vi "Draw Shapes.vi"(0 "Picture in":refnum<vi>, 1 "Commands":cluster{"Time (s)":dbl, T2, "Enabled":bool}[](array[cluster]), 2 "dt array":dbl[](array[numeric]), 3 "Sample Period (s)":dbl=0.02, 5 "Points":cluster{"x":dbl, "y":dbl, "th":dbl}[](array[cluster]), 7 "new picture in":picture, 9 "Path Type":T1, 11 "Results":T5, 12 "Output Point":T4, 14 "Path Points":cluster{"x":dbl, "y":dbl}[](array[cluster])) -> (4 "new picture out":picture)   [LabVIEW 2025]
uses:
  Types/Single Cmd Info.ctl
  <vilib>/picture/picture.llb/imagedata.ctl
  Types/Path Type.ctl
  Global Settings.vi
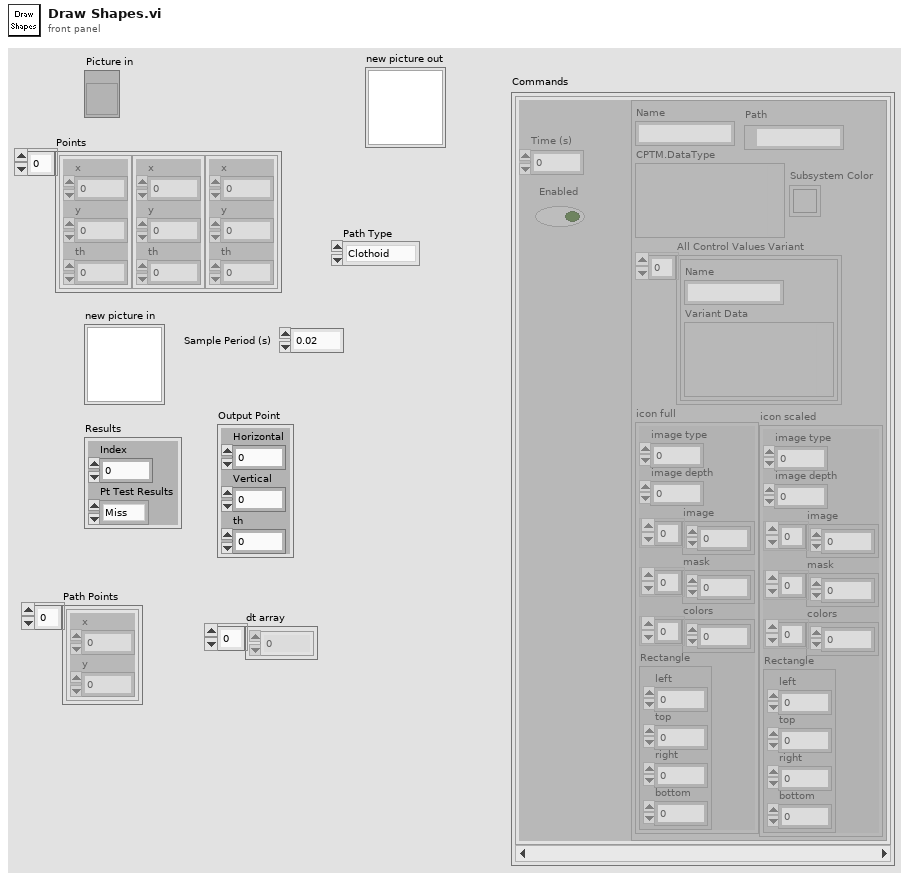
[diagram p1: front panel]
types:
  T1 = typedef "Path Type.ctl" = enum16{"Clothoid", "Bezier", "Choreo"}
  T2 = typedef "Single Cmd Info.ctl" = cluster{"Name":string, "CPTM.DataType":variant, "All Control Values Variant":cluster{"Name":string, "Variant Data":variant}[], "icon full":T3, "icon scaled":T3, "Path":path, "Subsystem Color":u32}
  T3 = typedef "imagedata.ctl" = cluster{"image type":i32, "image depth":i32, "image":u8[], "mask":u8[], "colors":u32[], "Rectangle":cluster{"left":i16, "top":i16, "right":i16, "bottom":i16}}
  T4 = cluster{"Horizontal":dbl, "Vertical":dbl, "th":dbl}
  T5 = cluster{"Index":i32, "Pt Test Results":enum16{"Miss", "Rect Hit", "Arrow Hit"}}
  T6 = typedef "LVPositionTypeDef.ctl" = cluster{"Left":i32, "Top":i32}
  T7 = typedef "LVBoundsTypeDef.ctl" = cluster{"Width":u32, "Height":u32}
  T8 = cluster{"left":i16, "top":i16, "right":i16, "bottom":i16}
  T9 = cluster{"Horizontal":dbl, "Vertical":dbl, "Horizontal":dbl, "Vertical":dbl}
  T10 = cluster{i32, "Pt Test Results":enum16{"Miss", "Rect Hit", "Arrow Hit"}}
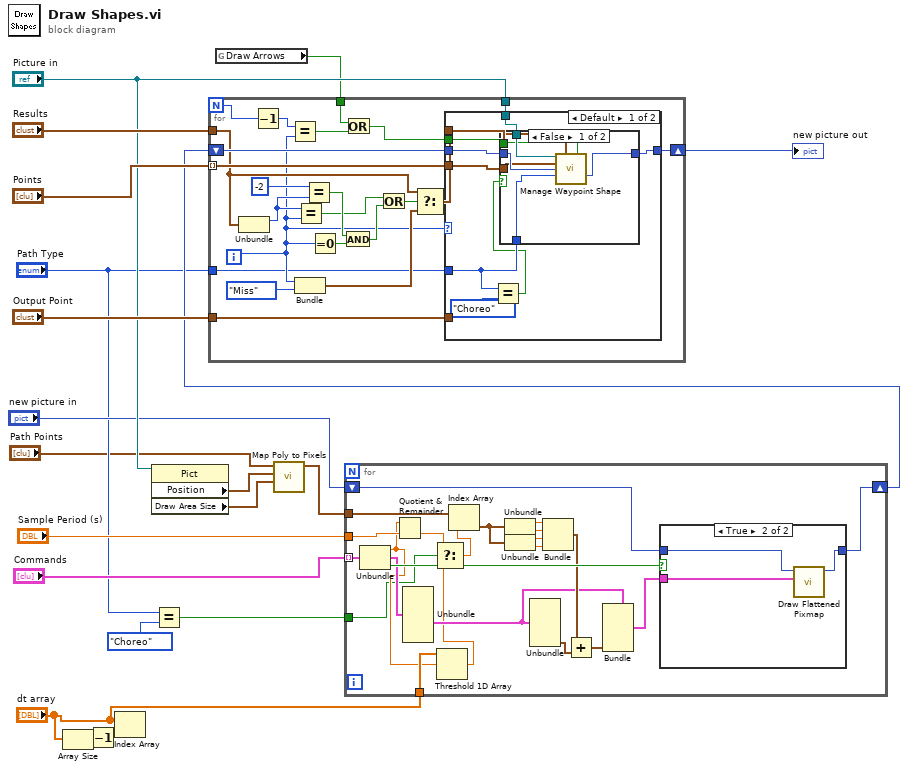
[diagram p0: block diagram]
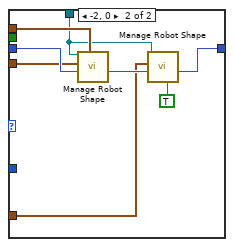
[diagram p4: hidden frame]
diagram:
  n1 = Array Size(array="dt array") -> (size(s)=w4:i32)
  n2 = Decrement(x=w4) -> (x-1=w3:i32)
  n3 = Index Array(array="dt array", index=w3) -> ()  [unwired: 1 out]
  n4 = property on="Property Node" class="Pict"(reference="Picture in") -> ("Position"=w14:T6, "Draw Area Size"=w15:T7)  [unwired: 1 in, 2 out]
  n5 = Equal?(x="Path Type", y=Path_Type."Choreo") -> (x = y?=w1:bool)
  n6 = global read "Global Settings.vi" "Draw Arrows"() -> (w8:bool)
  n7 = call "Map Poly to Pixels.vi"("Draw Area Size"=w15, "Position"=w14, "Coords"="Path Points") -> ("Coords"=w13:cluster{"Horizontal":dbl, "Vertical":dbl}[])  [unwired: 8 in]
  n8 = for {
    shift-right: [w38] -> w10
    shift-left: "new picture in" -> [w40]
    tunnel: "Commands" -> [w43] mode=indexing
    tunnel: w13 -> [w42]
    tunnel: "Sample Period (s)" -> [w41]
    tunnel: "dt array" -> [w26]
    tunnel: w1 -> [w24]
    n9 = Unbundle(w43) -> ("Time (s)"=w25:dbl, w36:T2, "Enabled"=w39:bool)
    n10 = Quotient & Remainder(x=w25, y=w41) -> (floor(x/y)=w23:dbl)  [unwired: 1 out]
    n11 = Unbundle(w36) -> ("icon scaled"=w28:T3)  [unwired: 6 out]
    n12 = Threshold 1D Array(2:w25, 3:w26) -> (0:w22:dbl)  [unwired: 1 in]
    n13 = Select(t=w22, s=w24, f=w23) -> (s? t:f=w21:dbl)
    n14 = Index Array(array=w42, index=w21) -> (element=w27:cluster{"Horizontal":dbl, "Vertical":dbl})
    n15 = Unbundle(w27) -> ("Horizontal"=w35:dbl, "Vertical"=w34:dbl)
    n16 = Unbundle(w27) -> ("Horizontal"=w33:dbl, "Vertical"=w32:dbl)
    n17 = Unbundle(w28) -> ("Rectangle"=w30:T8)  [unwired: 5 out]
    n18 = Bundle("Horizontal"=w35, "Vertical"=w34, "Horizontal"=w33, "Vertical"=w32) -> (w29:T9)  [unwired: 1 in]
    n19 = Add(x=w29, y=w30) -> (x+y=w37:cluster{dbl, dbl, dbl, dbl})
    n20 = Bundle(cluster=w28, "Rectangle"=w37) -> (w31:T3)  [unwired: 5 in]
    n21 = case shown="True" w39 {
      tunnel: [w44 w45] -> w38
      tunnel: w40 -> [w44 w46]
      tunnel: w31 -> [_ w47]
      frame False {
      }
      frame True {
        n22 = call <vilib>:"Draw Flattened Pixmap.vi"("image data"=w47, "picture"=w46) -> ("new picture"=w45:picture)  [unwired: 7 in]
      }
    }
  }
  n23 = for {
    N -> [w55]
    tunnel: "Points" -> [w70] mode=indexing
    shift-right: [w69] -> w9
    shift-left: w10 -> [w68]
    tunnel: "Picture in" -> [w67]
    tunnel: "Results" -> [w64]
    tunnel: "Output Point" -> [w52]
    tunnel: w8 -> [w49]
    tunnel: "Path Type" -> [w48]
    i -> [w53]
    n24 = Unbundle(w64) -> ("Index"=w60:i32)  [unwired: 1 out]
    n25 = Decrement(x=w55) -> (x-1=w54:i32)
    n26 = Equal?(x=w54, y=w53) -> (x = y?=w51:bool)
    n27 = Bundle(w53, "Pt Test Results"=enum16{"Miss", "Rect Hit", "Arrow Hit"}."Miss") -> (w65:T10)  [unwired: 1 in]
    n28 = Equal?(x=w60, y=w53) -> (x = y?=w57:bool)
    n29 = Equal?(x=-2, y=w60) -> (x = y?=w59:bool)
    n30 = Equal To 0?(x=w53) -> (x = 0?=w62:bool)
    n31 = And(x=w59, y=w62) -> (x .and. y?=w58:bool)
    n32 = Or(x=w49, y=w51) -> (x .or. y?=w50:bool)
    n33 = Or(x=w57, y=w58) -> (x .or. y?=w56:bool)
    n34 = Select(t=w64, s=w56, f=w65) -> (s? t:f=w66:T5)
    n35 = case shown="Default" w53 {
      tunnel: w70 -> [w75 w88]
      tunnel: [w78 w92] -> w69
      tunnel: w68 -> [w79 w95]
      tunnel: w67 -> [w77 w91]
      tunnel: w66 -> [w76 w94]
      tunnel: w50 -> [w74 _]
      tunnel: w52 -> [_ w89]
      tunnel: w48 -> [w73 _]
      frame Default {
        n36 = Equal?(x=w73, y=Path_Type."Choreo") -> (x = y?=w71:bool)
        n37 = case shown="False" w71 {
          tunnel: w79 -> [w86 w87]
          tunnel: [w85 w87] -> w78
          tunnel: w77 -> [w84 _]
          tunnel: w76 -> [w83 _]
          tunnel: w75 -> [w82 _]
          tunnel: w74 -> [w81 _]
          tunnel: w73 -> [w80 _]
          frame False {
            n38 = call "Manage Waypoint Shape.vi"("Pict Ref"=w84, "Drawing Options"=w83, "Draw Arrow"=w81, "Waypoint Position (ft)"=w82, "new picture in"=w86, "Path Type"=w80) -> ("new picture out"=w85:picture)  [unwired: 8 in, 1 out]
          }
          frame True {
          }
        }
      }
      frame -2, 0 {
        n39 = call "Manage Robot Shape.vi"("Drawing Options"=w94, "new picture in"=w95, "Robot Position (ft)"=w88, "Pict Ref"=w91) -> ("new picture out"=w93:picture)  [unwired: 5 in, 2 out]
        n40 = call "Manage Robot Shape.vi"("Lighter"=TRUE ("Outline"), "new picture in"=w93, "Robot Position (ft)"=w89, "Pict Ref"=w91) -> ("new picture out"=w92:picture)  [unwired: 5 in, 2 out]
      }
    }
  }
  "new picture out" <- w9
